vi "Pipe Viscometer #2.vi"() -> ()   [LabVIEW 2017]
uses:
  Flow Out PVisco.vi
  Flow Set PVisco.vi
  Halt PVisco.vi
  <vilib>/addons/control/pid/pid.llb/PID Control Input Filter (DBL).vi
  <vilib>/addons/control/pid/pid.llb/PID Advanced (DBL).vi
  <vilib>/addons/control/pid/NI_PID_pid.lvlib
panel:
  out "Pressure Drop (small pipe)":dbl caption="\"WC" format="%.1f"
  in  "Pump Switch":bool
  out "Fluid Temperature":dbl format="%.1f"
  out "Liquid Flowrate":dbl format="%.1f"
  in  "Flowrate Setpoint":dbl=40.0 caption="gal/min" format="%.1f"
  out "% Pump Speed":dbl(slide) scale=0.0..100.0
  in  "Manual Control Override":bool=TRUE
  in  "Set Manual % Pump Speed":dbl(slide)=49.494949494949495 scale=0.0..100.0
  in  "stop":bool
  in  "Kc":dbl=1.0
  in  "Ti":dbl=0.05 caption="(min)"
  in  "Td":dbl caption="(min)"
  out "Data Point Count":i32
  in  "Specify Time between Data Points (sec)":dbl=1.0
  in  "Cancel Data Collection":bool
  in  "Specify number of data points":i16=1
  in  "Enable 4":bool
  out "Saving Data 4":bool
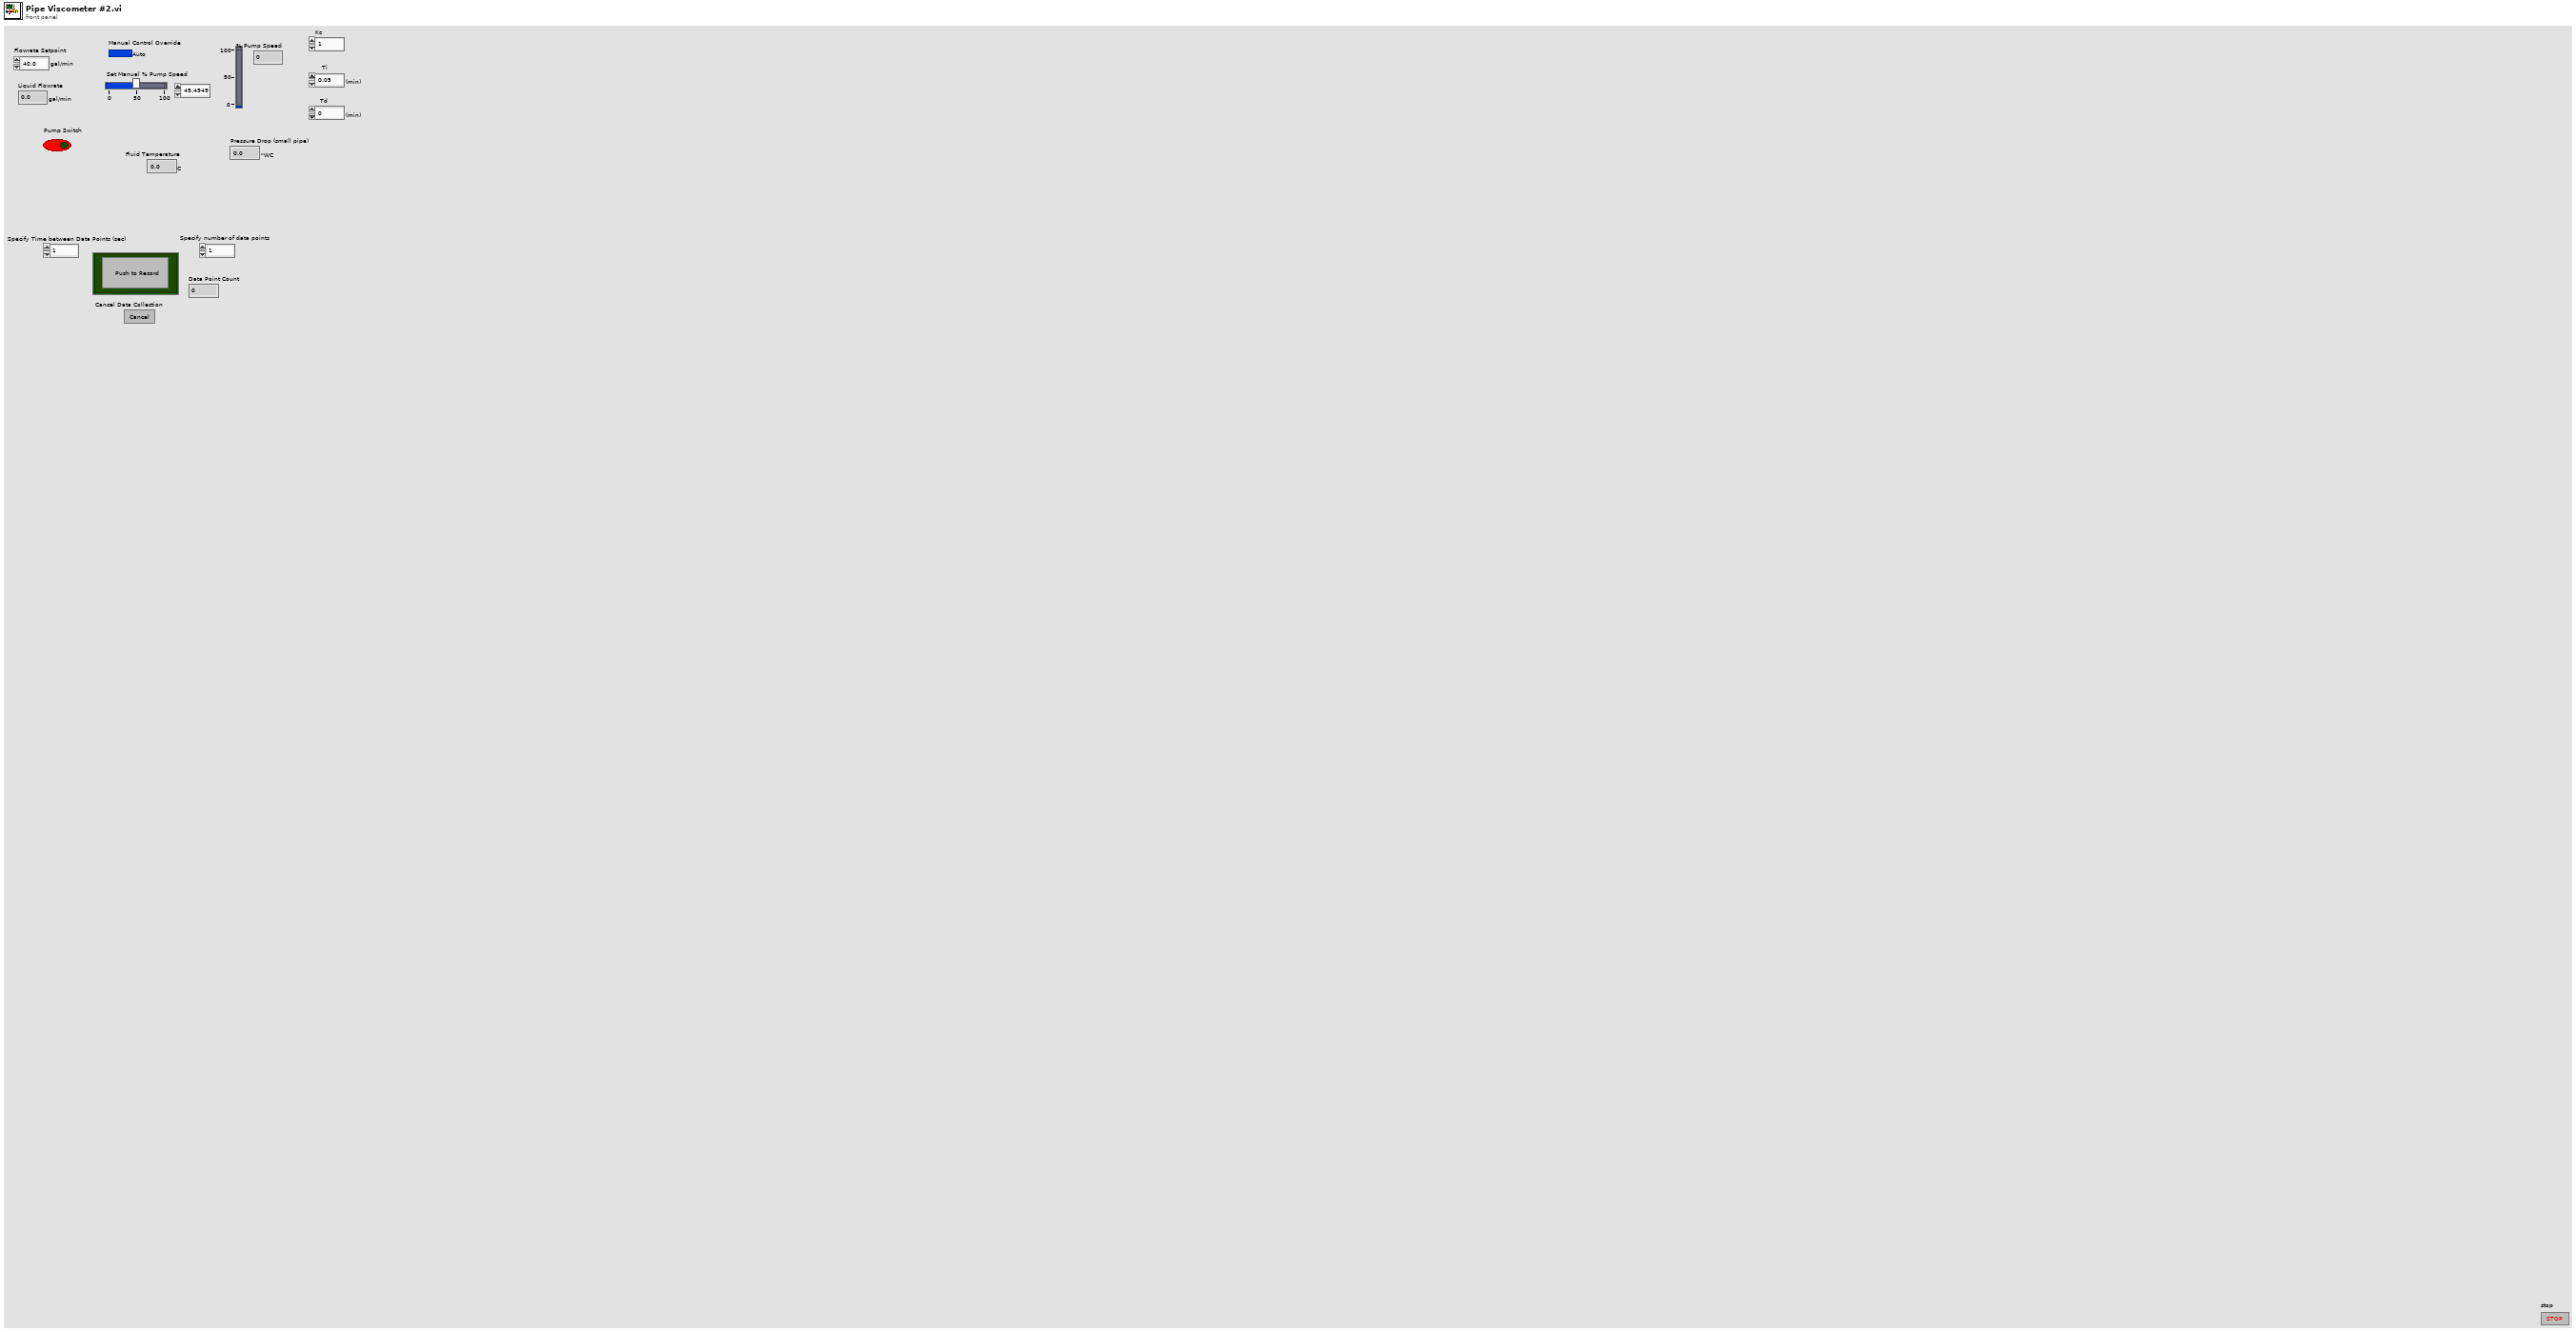
[diagram p1: front panel]
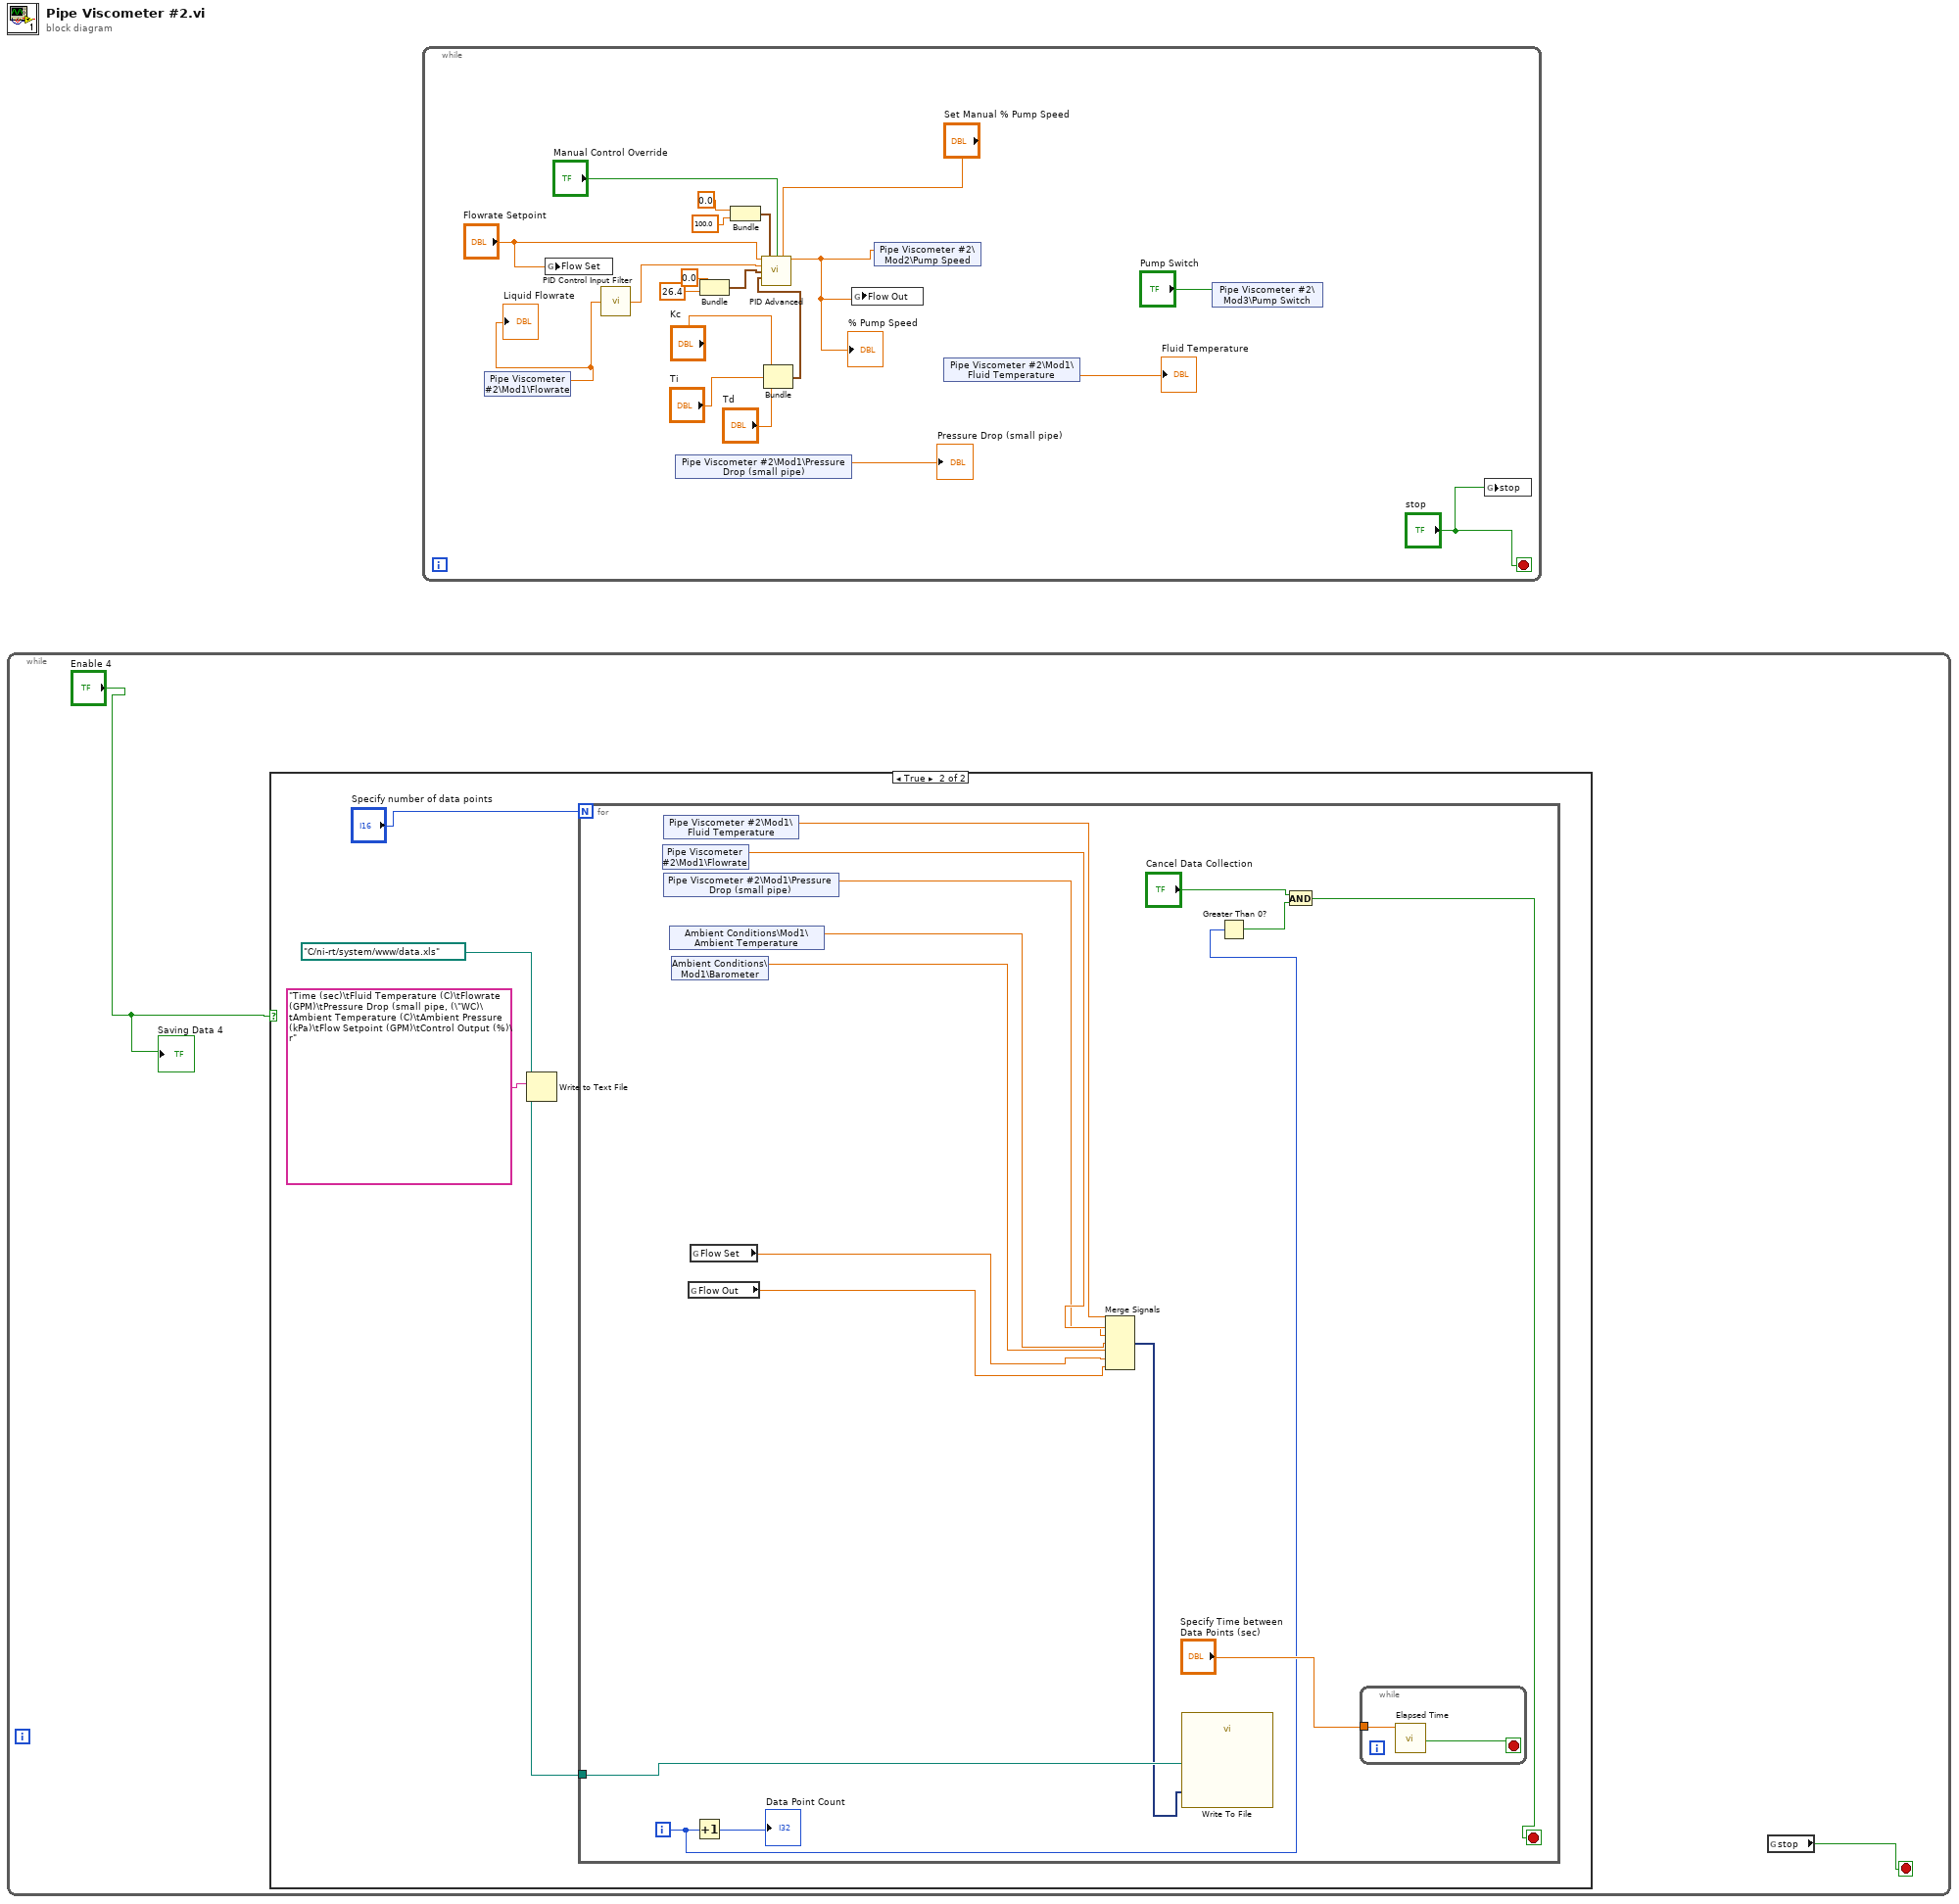
[diagram p0: block diagram]
diagram:
  n1 = while {
    stop <- w1 stop-if-true
    n2 = case shown="True" "Enable 4" {
      frame False {
      }
      frame True {
        w4 = path "C:/ni-rt/system/www/data.xls" ("Filename")
        n3 = Write to Text File(file (use dialog)=w4, text="Time (sec)\tFluid Temperature (C)\tFlowrate (GPM)\tPressure Drop (small pipe, (\"WC)\tAmbient Temperature (C)\tAmbient Pressure (kPa)\tFlow Setpoint (GPM)\tControl Output (%)\r") -> ()  [unwired: 2 in, 3 out]
        n4 = for {
          N: "Specify number of data points" -> [_]
          tunnel: w4 -> [w20]
          i -> [w14]
          stop <- w11 stop-if-true
          n5 = shared-variable "Pipe Viscometer #2\\Mod1\\Flowrate"() -> (w17:dbl)  [unwired: 1 in, 1 out]
          n6 = shared-variable "Pipe Viscometer #2\\Mod1\\Fluid Temperature"() -> (w18:dbl)  [unwired: 1 in, 1 out]
          n7 = shared-variable "Pipe Viscometer #2\\Mod1\\Pressure Drop (small pipe)"() -> (w10:dbl)  [unwired: 1 in, 1 out]
          n8 = shared-variable "Ambient Conditions\\Mod1\\Ambient Temperature"() -> (w9:dbl)  [unwired: 1 in, 1 out]
          n9 = shared-variable "Ambient Conditions\\Mod1\\Barometer"() -> (w8:dbl)  [unwired: 1 in, 1 out]
          n10 = global read "Flow Out PVisco.vi" "Flow Out"() -> (w6:dbl)
          n11 = global read "Flow Set PVisco.vi" "Flow Set"() -> (w7:dbl)
          n12 = Increment(x=w14) -> (x+1=→"Data Point Count":i32)
          n13 = Merge Signals(w18, w17, w10, w9, w8, w7, w6) -> (w16:dynamicdata)
          n14 = call "Write To File"("Signals"=w16, "Filename"=w20) -> ()  [unwired: 15 in, 3 out]
          n15 = Greater Than 0?(x=w14) -> (x > 0?=w12:bool)
          n16 = And(x="Cancel Data Collection", y=w12) -> (x .and. y?=w11:bool)
          n17 = while {
            tunnel: "Specify Time between Data Points (sec)" -> [w21]
            stop <- w22 stop-if-true
            n18 = call "Elapsed Time"("Time Target (s)"=w21) -> ("Time has Elapsed"=w22:bool)  [unwired: 11 in, 7 out]
          }
        }
      }
    }
    n19 = global read "Halt PVisco.vi" "stop"() -> (w1:bool)
    "Saving Data 4" <- "Enable 4"
  }
  n20 = while {
    stop <- "stop" stop-if-true
    n21 = shared-variable "Pipe Viscometer #2\\Mod1\\Flowrate"() -> (w24:dbl)  [unwired: 1 in, 1 out]
    "Liquid Flowrate" <- w24
    n22 = global write "Flow Set PVisco.vi" "Flow Set"("Flowrate Setpoint") -> ()
    n23 = call-poly <vilib>:"PID Control Input Filter.vi"("input"=w24) -> ("output"=w23:dbl)  [unwired: 4 in]
    n24 = shared-variable "Pipe Viscometer #2\\Mod1\\Pressure Drop (small pipe)"() -> (→"Pressure Drop (small pipe)":dbl)  [unwired: 1 in, 1 out]
    n25 = Bundle(0.0, 26.4) -> (w25:cluster{dbl, dbl})  [unwired: 1 in]
    n26 = Bundle(0.0, 100.0) -> (w28:cluster{dbl, dbl})  [unwired: 1 in]
    n27 = Bundle("Kc"="Kc", "Ti"="Ti", "Td"="Td") -> (w42:cluster{"Kc":dbl, "Ti":dbl, "Td":dbl})  [unwired: 1 in]
    n28 = call-poly <vilib>:"PID Advanced.vi"("setpoint"="Flowrate Setpoint", "output range"=w28, "auto? (T)"="Manual Control Override", "manual control"="Set Manual % Pump Speed", "process variable"=w23, "setpoint range"=w25, "PID gains"=w42) -> ("output"=w32:dbl)  [unwired: 7 in, 1 out]
    "% Pump Speed" <- w32
    n29 = global write "Flow Out PVisco.vi" "Flow Out"(w32) -> ()
    n30 = shared-variable "Pipe Viscometer #2\\Mod2\\Pump Speed"(w32) -> ()  [unwired: 1 in, 1 out]
    n31 = shared-variable "Pipe Viscometer #2\\Mod1\\Fluid Temperature"() -> (→"Fluid Temperature":dbl)  [unwired: 1 in, 1 out]
    n32 = shared-variable "Pipe Viscometer #2\\Mod3\\Pump Switch"("Pump Switch") -> ()  [unwired: 1 in, 1 out]
    n33 = global write "Halt PVisco.vi" "stop"("stop") -> ()
  }
